vi "PID Discrete Controller.vi"() -> ()   [LabVIEW 2020]
uses:
  <vilib>/MakerHub/LINX/Public/Peripherals/Analog/Analog Read 1 Chan.vi
  <vilib>/MakerHub/LINX/Private/Local IO/LinxI2cWrite.vi
  <vilib>/MakerHub/LINX/Public/Utilities/Check Channel.vi
  <vilib>/MakerHub/LINX/Public/Peripherals/Analog/Analog Read N Chans.vi
  <vilib>/MakerHub/LINX/Private/Local IO/LinxAnalogRead.vi
  <vilib>/MakerHub/LINX/Public/Utilities/Open Serial.vi
  <vilib>/MakerHub/LINX/Private/Utilties/Generate Error.vi
  <vilib>/MakerHub/LINX/LMH-LINX.lvlib
panel:
  out "Salida":dynamicdata(graph)
  out "Señal de control":dbl(graph)
  out "r":dbl
  out "T":dbl
  out "IT":i32
  in  "SET":bool
  in  "Ref":dbl(slide) min=0.0 max=5.0 step=0.5 scale=0.0..5.0
  out "Error":dbl(graph)
  in  "tsim":dbl
  # "U(z)\n----\nE(z)"
  # "8.281e-05 + 0.0001656 z^-1 + 8.281e-05 z^-2\n  -------------------------------------------\n                          0.02 - 0.02 z^-1"
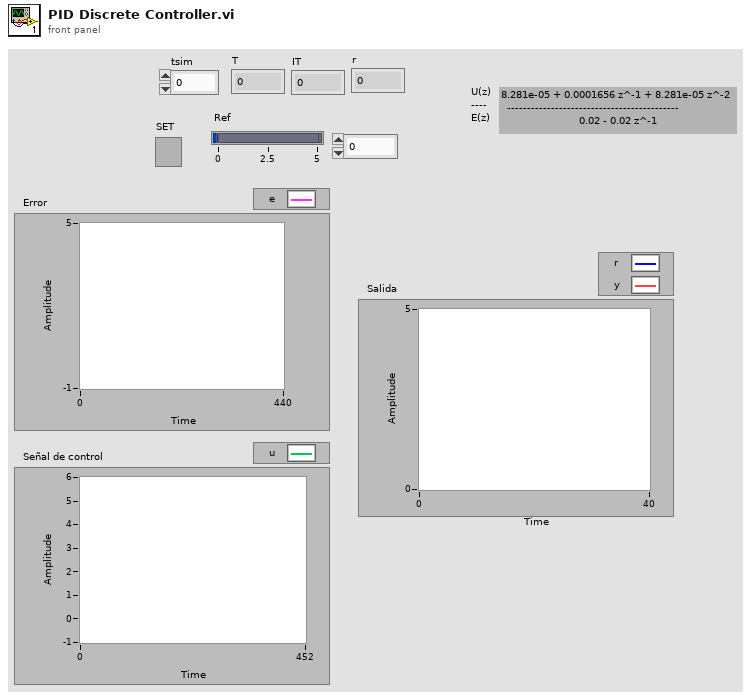
[diagram p1: front panel]
types:
  T1 = typedef "LMH-LINX.lvlib/LINX Ref.ctl" = cluster{"IO":T2, "Interface":T3, "LINX Device Config":T4}
  T2 = typedef "LMH-LINX.lvlib/Platform.ctl" = enum16{"Remote", "Local"}
  T3 = typedef "LMH-LINX.lvlib/Interface.ctl" = enum16{"Serial", "TCP"}
  T4 = typedef "LMH-LINX.lvlib/Device.lvlib/LINX Device Config.ctl" = cluster{"Interface":T3, "COM Port":refnum<visa-resource-name>, "TCP Configuration":T5, "Device Family":u8, "Device ID":u8, "Device Name":string, "TCP Ref":refnum<k5>, "Channels":T6}
  T5 = typedef "LMH-LINX.lvlib/Device.lvlib/TCP Config.ctl" = cluster{"IP Address":string, "Port":u16}
  T6 = typedef "LMH-LINX.lvlib/Channels.ctl" = cluster{"DI":u8[], "DO":u8[], "AI":u8[], "AO":u8[], "PWM":u8[], "QE":u8[], "UART":u8[], "I2C 2":u8[], "SPI":u8[], "CAN":u8[], "Servo":u8[], "AI Ref (V)":dbl, "AI Resolution (Bits)":u8, "AO Ref (V)":dbl, "AO Resolution (Bits)":u8}
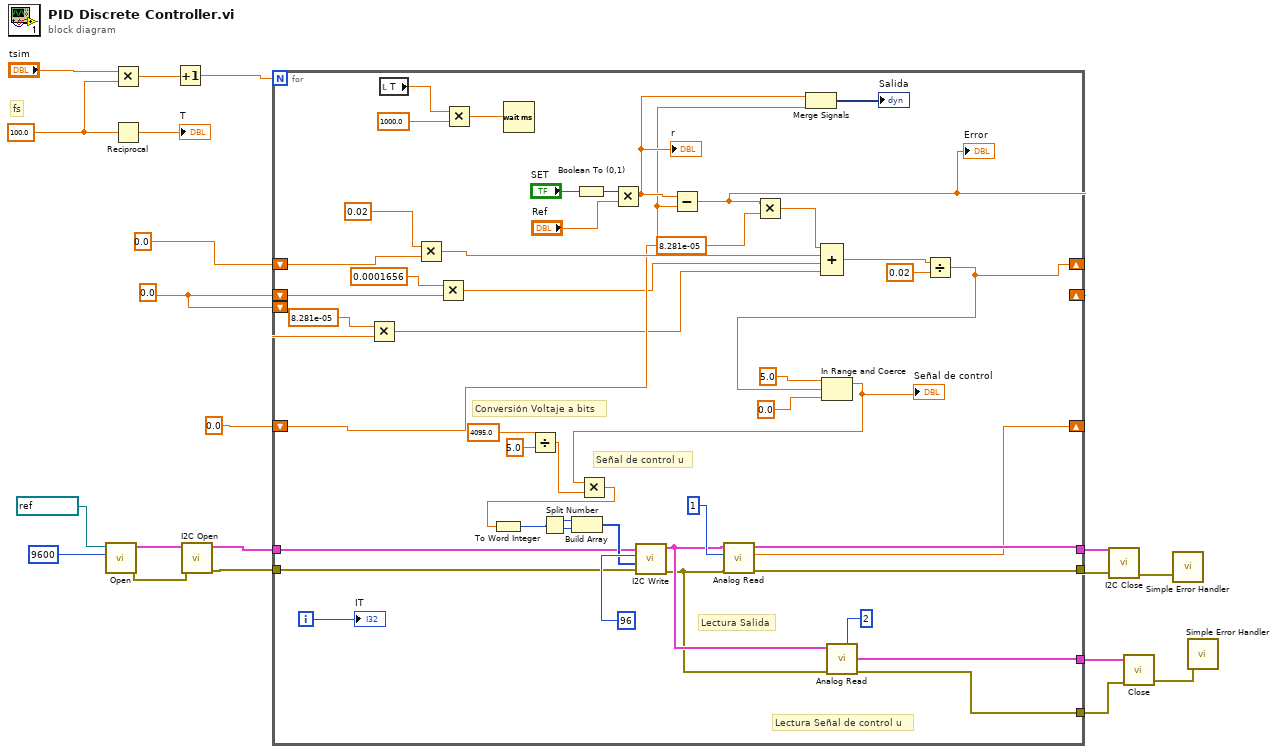
[diagram p0: block diagram]
diagram:
  w17 = 100.0 ("y")
  w1 = 0.0
  # "fs"
  n1 = call-poly <vilib>:"Open.vi"("Baud Rate Override"=u32 9600, "Serial Port"=refnum<visa-resource-name> "COM5") -> ("Error Out"=w12:errorcluster, "LINX Resource"=w13:T1)  [unwired: 7 in, 1 out]
  n2 = Multiply(x="tsim", y=w17) -> (x*y=w20:dbl)
  n3 = Reciprocal(x=w17) -> (1/x=→"T":dbl)
  n4 = Increment(x=w20) -> (x+1=w19:dbl)
  n5 = call <vilib>:"I2C Open.vi"("Error In"=w12, "LINX Resource"=w13) -> ("Error Out"=w4:errorcluster, "LINX Resource"=w5:T1)  [unwired: 8 in]
  n6 = for {
    N: w19 -> [_]
    shift-right: [w25] -> _
    shift-left: 0.0 -> [w33]
    shift-right: [w27] -> _
    shift-left: w1 -> [w38]
    shift-right: [w37] -> _
    shift-left: 0.0 ("Voltage") -> [w36]
    tunnel: w5 -> [w35]
    tunnel: [w42] -> w10
    tunnel: w4 -> [w34]
    tunnel: [w41] -> w9
    tunnel: [w29] -> w3
    tunnel: [w28] -> w2
    shift-left: w1 -> [w22]
    i -> [w65]
    # "Conversión Voltaje a bits"
    # "Señal de control u"
    # "Lectura Señal de control u"
    # "Lectura Salida"
    n7 = Multiply(x=8.281e-05, y=w22) -> (x*y=w21:dbl)
    n8 = local read "T"() -> (w68:dbl)
    n9 = Multiply(x=0.02, y=w33) -> (x*y=w58:dbl)
    n10 = Multiply(x=0.0001656, y=w38) -> (x*y=w24:dbl)
    n11 = Multiply(x=w68, y=1000.0) -> (x*y=w66:dbl)
    n12 = Wait (ms)(milliseconds to wait=w66) -> ()  [unwired: 1 out]
    n13 = Divide ("Divide 2")(x=4095.0 ("Constant"), y=5.0 ("y 2")) -> (x/y=w48:dbl)
    n14 = Boolean To (0,1)(Boolean="SET") -> (0, 1=w63:i16)
    n15 = Multiply(x=w63, y="Ref") -> (x*y=w40:dbl)
    "r" <- w40
    n16 = Subtract(x=w40, y=w36) -> (x-y=w27:dbl)
    "Error" <- w27
    n17 = Multiply(x=w27, y=8.281e-05) -> (x*y=w26:dbl)
    n18 = Merge Signals(w40, w36) -> (→"Salida":dynamicdata)
    n19 = Compound Arithmetic op=ADD(w26, w58, w24, w21) -> (w57:dbl)
    n20 = Divide(x=w57, y=0.02) -> (x/y=w25:dbl)
    n21 = In Range and Coerce(upper limit=5.0, x=w25, lower limit=0.0) -> (coerced(x)=w30:dbl)  [unwired: 1 out]
    "Señal de control" <- w30
    n22 = Multiply(x=w30, y=w48) -> (x*y=w47:dbl)
    n23 = To Word Integer(number=w47) -> (16bit integer=w51:i16)
    n24 = Split Number(x=w51) -> (hi(x)=w50:u8, lo(x)=w49:u8)
    n25 = Build Array ("Build Array 4")(w50, w49) -> (w46:u8[])
    n26 = call <vilib>:"I2C Write.vi"("Error In"=w34, "Data"=w46, "I2C Slave Address (0)"=u8 96, "LINX Resource"=w35) -> ("Error Out"=w43:errorcluster, "LINX Resource"=w44:T1)  [unwired: 6 in]
    n27 = call-poly <vilib>:"Analog Read.vi"("Error In"=w43, "Analog Channel"=u8 1 ("AO Channel"), "LINX Resource"=w44) -> ("Error Out"=w41:errorcluster, "Voltage"=w37:dbl, "LINX Resource"=w42:T1)  [unwired: 5 in, 1 out]
    n28 = call-poly <vilib>:"Analog Read.vi"("Error In"=w43, "Analog Channel"=u8 2, "LINX Resource"=w44) -> ("Error Out"=w28:errorcluster, "LINX Resource"=w29:T1)  [unwired: 5 in, 2 out]
    "IT" <- w65
  }
  n29 = call <vilib>:"I2C Close.vi"("Error In"=w9, "LINX Resource"=w10) -> ("Error Out"=w11:errorcluster)  [unwired: 8 in, 1 out]
  n30 = call <vilib>:"Close.vi"("Error In"=w2, "LINX Resource"=w3) -> ("Error Out"=w8:errorcluster)  [unwired: 9 in]
  n31 = call <vilib>:"Simple Error Handler.vi"("error in (no error)"=w11) -> ()  [unwired: 4 in, 5 out]
  n32 = call <vilib>:"Simple Error Handler.vi"("error in (no error)"=w8) -> ()  [unwired: 4 in, 5 out]
